vi "write_table_mode_command_v3.vi"(10 "Synth Controls":T1={"Channel Settings"=[{"Voltage (Amp.) "=0.0, "Frequency (MHz)"=0.0, "Phase (deg)"=0.0, "Nickname"="Channel 0 D"}, {"Voltage (Amp.) "=0.0, "Frequency (MHz)"=0.0, "Phase (deg)"=0.0, "Nickname"="Channel 0 D"}, {"Voltage (Amp.) "=0.0, "Frequency (MHz)"=0.0, "Phase (deg)"=0.0, "Nickname"="Channel 0 D"}, {"Voltage (Amp.) "=0.0, "Frequency (MHz)"=0.0, "Phase (deg)"=0.0, "Nickname"="Channel 0 D"}], "Active Chans"=[TRUE, FALSE, FALSE, FALSE], "COM Port"="COM5", "Table Mode"={"Initial Freq.(MHz)"=0.0, "FinalFreq"=0.0, "Freq. Step (MHz)"=0.0, "Voltage (Amp.)"=1.0, "Asc. & Desc."=FALSE, "Custom Frequencies"=[], "Custom Amplitude"=[], "Table Mode Switch"=FALSE, "Array Gen"=enum."Auto", "Randomize"=FALSE, "Continuous"=FALSE}} {"Table Mode"."Freq. Step (MHz)" format="%#_9g"; "Table Mode"."FinalFreq" format="%#_9g"; "Table Mode"."Initial Freq.(MHz)" format="%#_9g"; "Channel Settings"."Frequency (MHz)" format="%#_9g"}) -> (2 "Table Mode Command":string)   [LabVIEW 2016]
uses:
  Controls/Synth_409b/Synth_controls.ctl
  Controls/Synth_409b/synth_channel.ctl
  Controls/Synth_409b/table_mode.ctl
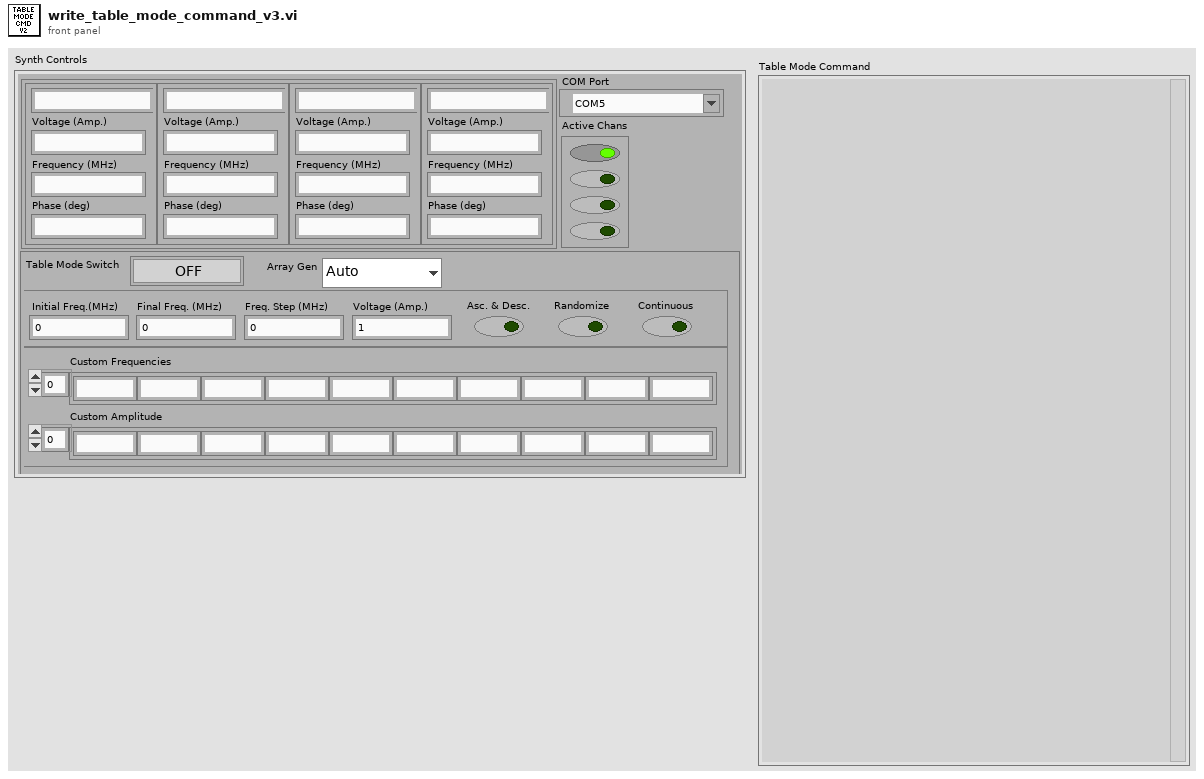
[diagram p1: front panel]
types:
  T1 = typedef "Synth_controls.ctl" = cluster{"Channel Settings":T2[], "Active Chans":bool[], "COM Port":refnum<visa-resource-name>, "Table Mode":T3}
  T2 = typedef "synth_channel.ctl" = cluster{"Voltage (Amp.) ":dbl, "Frequency (MHz)":dbl, "Phase (deg)":dbl, "Nickname":string}
  T3 = typedef "table_mode.ctl" = cluster{"Initial Freq.(MHz)":dbl, "FinalFreq":dbl, "Freq. Step (MHz)":dbl, "Voltage (Amp.)":dbl, "Asc. & Desc.":bool, "Custom Frequencies":dbl[], "Custom Amplitude":dbl[], "Table Mode Switch":bool, "Array Gen":enum16{"Auto", "Custom"}, "Randomize":bool, "Continuous":bool}
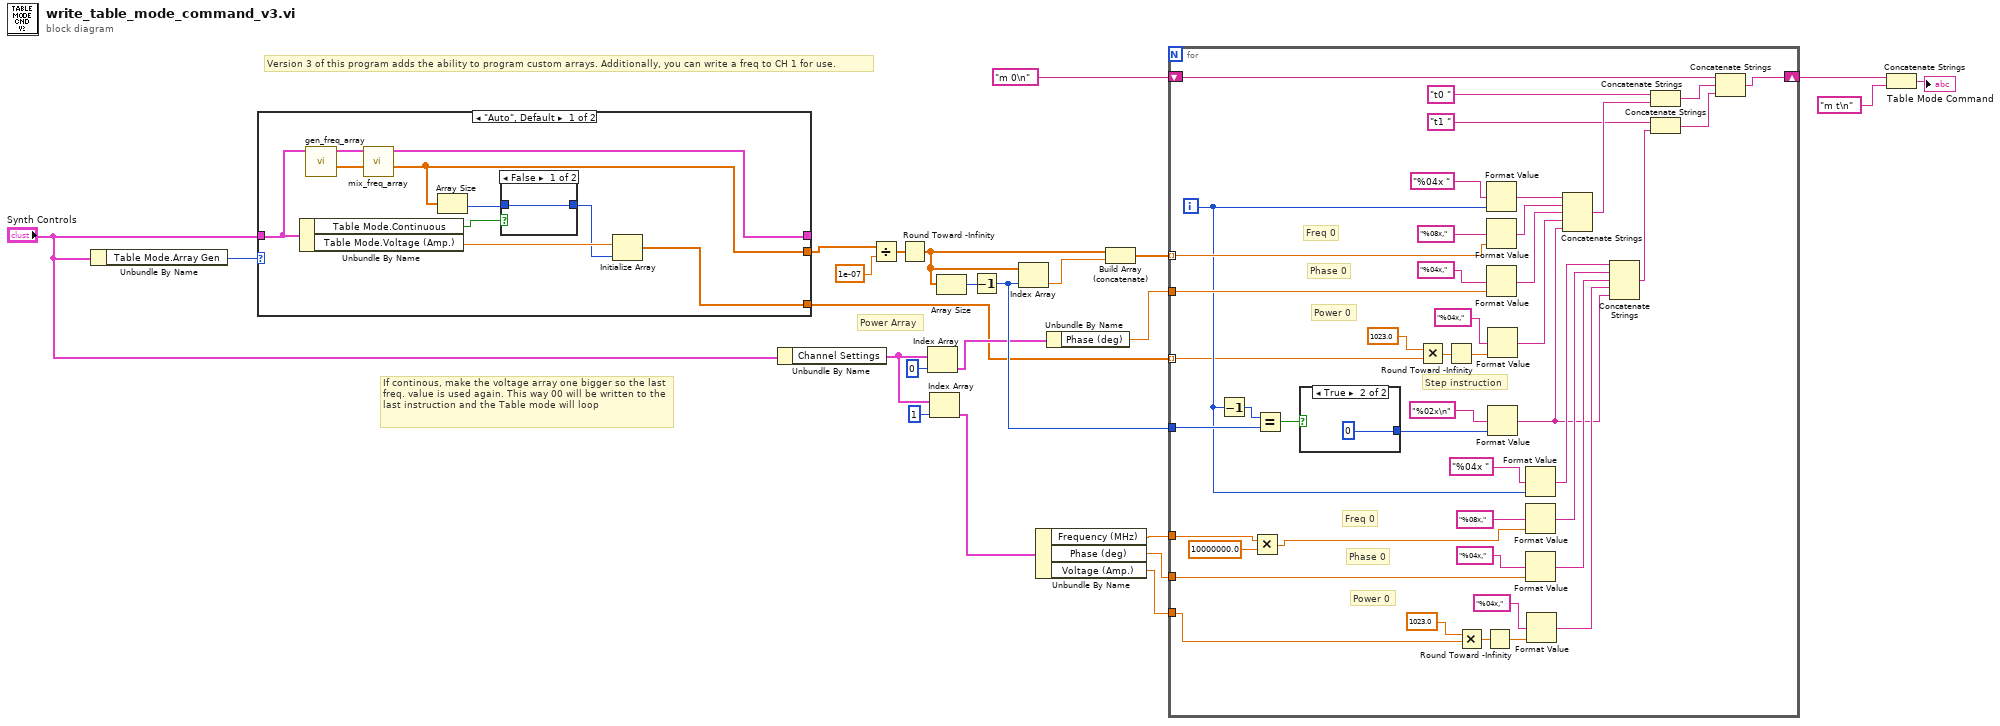
[diagram p0: block diagram]
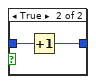
[diagram p2: hidden frame]
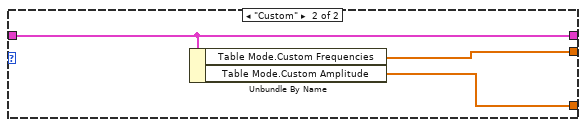
[diagram p3: hidden frame]
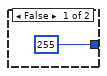
[diagram p4: hidden frame]
diagram:
  # "If continous, make the voltage array one bigger so the last freq. value is used again. This way 00 will be written to the last instruction and the Table mode will loop"
  # "Power Array"
  # "Version 3 of this program adds the ability to program custom arrays. Additionally, you can write a freq to CH 1 for use."
  n1 = Unbundle By Name("Synth Controls") -> ("Table Mode.Array Gen"=w3:enum16{"Auto", "Custom"})
  n2 = case shown="\"Auto\", Default" w3 {
    tunnel: [w28 w39] -> w1
    tunnel: [w29 w40] -> _
    tunnel: "Synth Controls" -> [w34 w40]
    tunnel: [w33 w38] -> w2
    frame "Auto", Default {
      n3 = Unbundle By Name(w34) -> ("Table Mode.Continuous"=w25:bool, "Table Mode.Voltage (Amp.)"=w32:dbl)
      n4 = call "gen_freq_array.vi"("Synth Controls"=w34) -> ("Synth Controls Out"=w30:T1, "Array"=w31:dbl[])  [unwired: 8 in]
      n5 = call "mix_freq_array.vi"("Freq Array In"=w31, "Synth Controls"=w30) -> ("Mixed Freq Array"=w28:dbl[], "Synth Controls Out"=w29:T1)  [unwired: 8 in]
      n6 = Array Size(array=w28) -> (size(s)=w27:i32)
      n7 = case shown="False" w25 {
        tunnel: w27 -> [w35 w37]
        tunnel: [w35 w36] -> w26
        frame False {
        }
        frame True {
          n8 = Increment(x=w37) -> (x+1=w36:i32)
        }
      }
      n9 = Initialize Array(w32, w26) -> (w33:dbl[])
    }
    frame "Custom" {
      n10 = Unbundle By Name(w40) -> ("Table Mode.Custom Frequencies"=w39:dbl[], "Table Mode.Custom Amplitude"=w38:dbl[])
    }
  }
  n11 = Unbundle By Name("Synth Controls") -> ("Channel Settings"=w9:T2[])
  n12 = Divide(x=w1, y=1e-07) -> (x/y=w22:dbl[])
  n13 = Round Toward -Infinity(1:w22) -> (0:w17:dbl[])
  n14 = Index Array(array=w9, index=0) -> (element=w12:T2)
  n15 = Index Array(array=w9, index=1) -> (element=w8:T2)
  n16 = Array Size(array=w17) -> (size(s)=w19:i32)
  n17 = Decrement(x=w19) -> (x-1=w15:i32)
  n18 = Index Array(array=w17, index=w15) -> (element=w18:dbl)
  n19 = Unbundle By Name(w8) -> ("Frequency (MHz)"=w7:dbl, "Phase (deg)"=w6:dbl, "Voltage (Amp.)"=w5:dbl)
  n20 = Unbundle By Name(w12) -> ("Phase (deg)"=w11:dbl)
  n21 = Build Array (concatenate)(w17, w18) -> (w16:dbl[])
  n22 = for {
    shift-right: [w77] -> w21
    shift-left: "m 0\n" -> [w76]
    tunnel: w16 -> [w83] mode=indexing
    tunnel: w15 -> [w70]
    tunnel: w11 -> [w61]
    tunnel: w7 -> [w43]
    tunnel: w6 -> [w46]
    tunnel: w5 -> [w47]
    tunnel: w2 -> [w41] mode=indexing
    i -> [w45]
    # "Power 0"
    # "Freq 0"
    # "Phase 0"
    # "Power 0"
    # "Freq 0"
    # "Step instruction"
    # "Phase 0"
    n23 = Decrement(x=w45) -> (x-1=w67:i32)
    n24 = Multiply(x=w43, y=10000000.0) -> (x*y=w42:dbl)
    n25 = Equal?(x=w67, y=w70) -> (x = y?=w69:bool)
    n26 = case shown="True" w69 {
      tunnel: [255 0] -> w68
      frame False {
      }
      frame True {
      }
    }
    n27 = Multiply(x=1023.0, y=w41) -> (x*y=w64:dbl)
    n28 = Round Toward -Infinity(1:w64) -> (0:w63:dbl)
    n29 = Multiply(x=1023.0, y=w47) -> (x*y=w52:dbl)
    n30 = Round Toward -Infinity(1:w52) -> (0:w51:dbl)
    n31 = Format Value(format string="%04x ", value (0)=w45) -> (output string=w84:string)  [unwired: 1 in]
    n32 = Format Value(format string="%08x,", value (0)=w83) -> (output string=w81:string)  [unwired: 1 in]
    n33 = Format Value(format string="%04x,", value (0)=w61) -> (output string=w79:string)  [unwired: 1 in]
    n34 = Format Value(format string="%04x,", value (0)=w63) -> (output string=w65:string)  [unwired: 1 in]
    n35 = Format Value(format string="%02x\n", value (0)=w68) -> (output string=w49:string)  [unwired: 1 in]
    n36 = Format Value(format string="%04x ", value (0)=w45) -> (output string=w59:string)  [unwired: 1 in]
    n37 = Format Value(format string="%08x,", value (0)=w42) -> (output string=w57:string)  [unwired: 1 in]
    n38 = Format Value(format string="%04x,", value (0)=w46) -> (output string=w55:string)  [unwired: 1 in]
    n39 = Format Value(format string="%04x,", value (0)=w51) -> (output string=w53:string)  [unwired: 1 in]
    n40 = Concatenate Strings(w84, w81, w79, w65, w49) -> (w75:string)
    n41 = Concatenate Strings(w59, w57, w55, w53, w49) -> (w48:string)
    n42 = Concatenate Strings("t0 ", w75) -> (w71:string)
    n43 = Concatenate Strings("t1 ", w48) -> (w72:string)
    n44 = Concatenate Strings(w76, w71, w72) -> (w77:string)
  }
  n45 = Concatenate Strings(w21, "m t\n") -> (→"Table Mode Command":string)
